vi "Test_NudgeUp_ValueDecrement.vi"(8 "error in (no error)":errorcluster, 11 "TestCase in":refnum<class "TestListboxExtensions.lvclass">) -> (0 "error out":errorcluster, 3 "TestCase in":refnum<class "TestListboxExtensions.lvclass">)   [LabVIEW 2015, in "TestListboxExtensions.lvclass"]
uses:
  TestListboxExtensions.lvclass
  <vilib>/addons/_JKI Toolkits/VI Tester/TestCase.llb/TestCase.lvclass
  ListboxExtensions.lvlib
panel:
  in  "Multicolumn Listbox":i32(listbox)
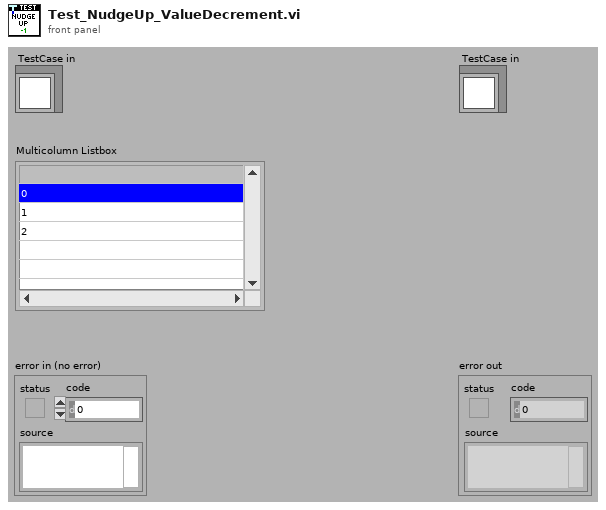
[diagram p1: front panel]
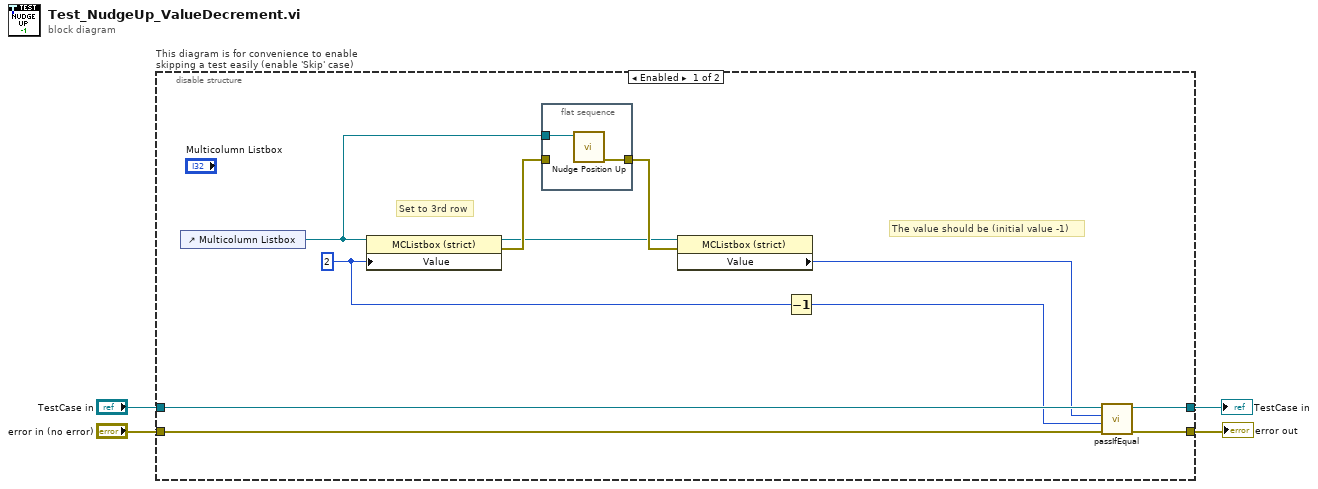
[diagram p0: block diagram]
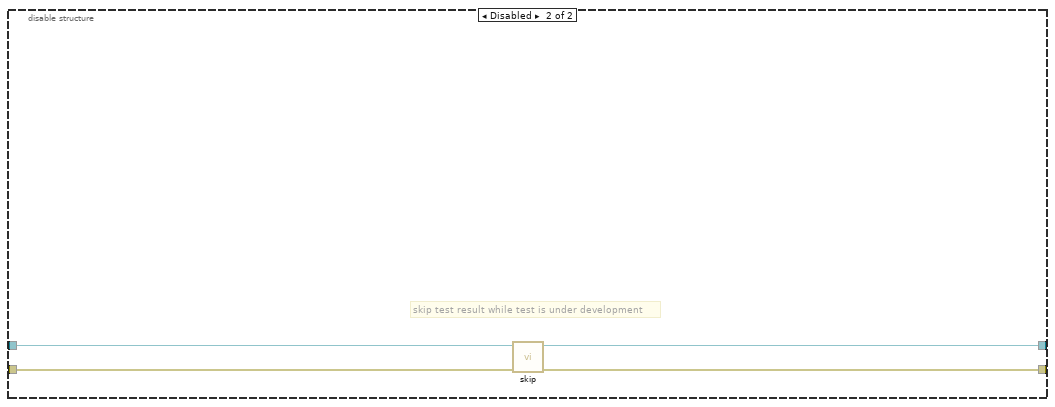
[diagram p2: hidden frame]
diagram:
  n1 = disable-structure "This diagram is for convenience to enable skipping a test easily (enable 'Skip' case)" shown="Enabled" {
    disable-tunnel: "TestCase in" -> [w15 w21]
    disable-tunnel: [w14 w19] -> w1
    disable-tunnel: [w13 w20] -> w3
    disable-tunnel: "error in (no error)" -> [w12 w18]
    frame Enabled {
      w10 = 2 ("Value")
      # "Set to 3rd row"
      # "The value should be (initial value -1)"
      n2 = control-ref of="Multicolumn Listbox"() -> (w5:refnum<vi>)
      n3 = property class="MCListbox (strict)"(reference=w5, "Value"=w10) -> (reference out=w6:refnum<vi>, error out=w7:errorcluster)  [unwired: 1 in]
      n4 = flat-sequence {
        tunnel: [w17] -> w11
        tunnel: w5 -> [w16]
        tunnel: w7 -> [_]
        frame #0 {
          n5 = call "Nudge Position Up.vi"("MulticolumnListbox in"=w16) -> ("error out"=w17:errorcluster)  [unwired: 10 in]
        }
      }
      n6 = property class="MCListbox (strict)"(reference=w6, error in=w11) -> ("Value"=w9:i32)  [unwired: 2 out]
      n7 = Decrement(x=w10) -> (x-1=w8:i32)
      n8 = call-dynamic "passIfEqual.vi"("error in (no error)"=w12, "y"=w8, "x"=w9, "TestCase in"=w15) -> ("error out"=w13:errorcluster, "TestCase out"=w14:refnum<class "TestListboxExtensions.lvclass">)  [unwired: 6 in]
    }
    frame Disabled {
      # "skip test result while test is under development"
      n9 = call <vilib>:"skip.vi"("error in (no error)"=w18, "TestCase in"=w21) -> ("error out"=w20:errorcluster, "TestCase out"=w19:refnum<class "TestListboxExtensions.lvclass">)  [unwired: 8 in]
    }
  }
  "error out" <- w3
  "TestCase in" <- w1
